vi "Begin.vi"(8 "error in":errorcluster) -> (0 "error out":errorcluster)   [LabVIEW 2017]
doc: "Called before other user functions, this VI is expected to open initial I/O refnums, load in file data, and do all program initialization. Notice that the <B>error out</B> terminal is simply used for data flow. Wiring it to other structures or subVIs ensures that this VI runs first."
uses:
  <vilib>/Rock Robotics/SystemInterfaces/DIO/FPGA_DIOPWMChannel.ctl
  <vilib>/Rock Robotics/WPI/SafetyOutput/WPI_SafetyOutputConfigMenu.ctl
  <vilib>/Rock Robotics/WPI/DriverStation/WPI_DriverStationRobotMode2.ctl
  <vilib>/Rock Robotics/WPI/Joystick/WPI_JoystickDeviceEnum.ctl
  <vilib>/Rock Robotics/SystemInterfaces/DIO/FPGA_DIOChannel.ctl
  <vilib>/Rock Robotics/SystemInterfaces/spilib/spi_bus.ctl
  <vilib>/Rock Robotics/WPI/RobotDrive/WPI_RobotDriveOpen2MotorWithVictorSP.vi
  Robot Global Data.vi
  <vilib>/Rock Robotics/Network Tables/NT Write String Array.vi
  <vilib>/Rock Robotics/WPI/Counter/WPI_CounterDigitalInputToDigitalSource.vi
  <vilib>/Rock Robotics/WPI/Gyro/WPI_GyroXRS450_SPI_Open.vi
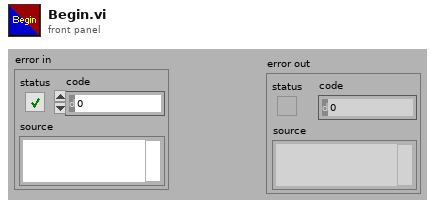
[diagram p1: front panel]
types:
  T1 = typedef "spi_bus.ctl" = enum16{"SPI On-Board, CS0", "SPI On-Board, CS1", "SPI On-Board, CS2", "SPI On-Board, CS3", "SPI MXP", "Invalid"}
  T2 = typedef "FPGA_DIOChannel.ctl" = enum8{"DIO 0", "DIO 1", "DIO 2", "DIO 3", "DIO 4", "DIO 5", "DIO 6", "DIO 7", "DIO 8", "DIO 9", "DIO MXP 0", "DIO MXP 1", "DIO MXP 2", "DIO MXP 3", "DIO MXP 4", "DIO MXP 5", "DIO MXP 6", "DIO MXP 7", "DIO MXP 8", "DIO MXP 9", "DIO MXP 10", "DIO MXP 11", "DIO MXP 12", "DIO MXP 13", "DIO MXP 14", "DIO MXP 15", "SPI Port CS1", "SPI Port CS2", "SPI Port CS3", "SPI Port MISO", "SPI Port MOSI", "Invalid"}
  T3 = typedef "WPI_JoystickDeviceEnum.ctl" = enum16{"USB 0", "USB 1", "USB 2", "USB 3", "USB 4", "USB 5"}
  T4 = typedef "WPI_DriverStationRobotMode2.ctl" = enum16{"Autonomous Disabled", "Autonomous Enabled", "Teleop Disabled", "Teleop Enabled", "Disconnected", "Finish", "Test Disabled", "Test Enabled", "Emergency Stopped"}
  T5 = typedef "WPI_SafetyOutputConfigMenu.ctl" = enum16{"Enable", "Disable"}
  T6 = typedef "FPGA_DIOPWMChannel.ctl" = enum8{"PWM 0", "PWM 1", "PWM 2", "PWM 3", "PWM 4", "PWM 5", "PWM 6", "PWM 7", "PWM 8", "PWM 9", "PWM MXP 0", "PWM MXP 1", "PWM MXP 2", "PWM MXP 3", "PWM MXP 4", "PWM MXP 5", "PWM MXP 6", "PWM MXP 7", "PWM MXP 8", "PWM MXP 9", "Invalid"}
  T7 = typedef "WPI_GyroDevRef.ctl" = cluster{"DevStatus":errorcluster, "Analog Channel":T8, "Gain (VoltsPerDegree/Second)":dbl, "Gyro Type":enum16{"Analog", "XRS450"}, "Handle":i32, "SPI Bus":T1, "Device Found":bool, "Sample Rate":dbl, "Calibrate On Open":bool, "Offset":dbl}
  T8 = typedef "FPGA_AIChannel.ctl" = enum8{"AI 0", "AI 1", "AI 2", "AI 3", "AI MXP 0", "AI MXP 1", "AI MXP 2", "AI MXP 3", "Invalid"}
  T9 = typedef "WPI_DigitalInputDevRef.ctl" = cluster{"DevStatus":errorcluster, "DIO Channel":T2}
  T10 = typedef "WPI_JoystickDevRef.ctl" = cluster{"Device":T3}
  T11 = typedef "WPI_RobotDriveDevRef.ctl" = cluster{"DevStatus":errorcluster, "Motors[]":T12[], "Square Inputs":bool, "Max Output":dbl}
  T12 = typedef "WPI_MotorControlDeviceRef.ctl" = cluster{"DeviceStatus":errorcluster, "Type":T13, "PWM":cluster{"PWM Channel":T6, "DeadBand":T14}, "CAN":cluster{"Device Number":u8, "SetOutput VI Ref":variant, "GetOutput VI Ref":variant, "Enable VI Ref":variant, "Disable VI Ref":variant, "Data":variant}, "Invert":bool, "DIO PWM":cluster{"PWM \"Enable\" Channel":T6, "DIOChannel":T2, "PWM Rate":dbl}}
  T13 = typedef "WPI_MotorControlType.ctl" = enum16{"PWM", "CAN", "DIO PWM"}
  T14 = typedef "WPI_PWMDeadband.ctl" = cluster{"Name":string, "maxPositivePwm":i32, "minPositivePwm":i32, "centerPwm":i32, "maxNegativePwm":i32, "minNegativePwm":i32, "angularRange":u16}
  T15 = typedef "FPGA_CounterEncoderSourceConvertionLVSourceType.ctl" = cluster{"DevStatus":errorcluster, "AnalogTriggerMode?":bool, "DigitalMode":cluster{"DIO Channel":T16}, "AnalogTriggerMode":cluster{"AnalogTriggerIndex":T17, "OutputType":T18}}
  T16 = typedef "FPGA_DIODigitalSourceChannel.ctl" = enum8{"DIO 0", "DIO 1", "DIO 2", "DIO 3", "DIO 4", "DIO 5", "DIO 6", "DIO 7", "DIO 8", "DIO 9", "DIO MXP 0", "DIO MXP 1", "DIO MXP 2", "DIO MXP 3", "DIO MXP 4", "DIO MXP 5", "DIO MXP 6", "DIO MXP 7", "DIO MXP 8", "DIO MXP 9", "DIO MXP 10", "DIO MXP 11", "DIO MXP 12", "DIO MXP 13", "DIO MXP 14", "DIO MXP 15", "Disabled"}
  T17 = typedef "FPGA_AnalogTriggerIndex.ctl" = enum8{"Trig 0", "Trig 1", "Trig 2", "Trig 3", "Trig 4", "Trig 5", "Trig 6", "Trig 7", "Invalid"}
  T18 = typedef "FPGA_AnalogTriggerOutType.ctl" = enum16{"InWindow", "TriggerState", "Rising", "Falling"}
  T19 = typedef "WPI_EncoderDevRef.ctl" = cluster{"DevStatus":errorcluster, "EncoderIndex":T20, "CounterIndex":T21, "DistancePerCount":dbl, "Decoding Type":T22}
  T20 = typedef "FPGA_EncoderIdx.ctl" = enum8{"Enc 0", "Enc 1", "Enc 2", "Enc 3", "Enc 4", "Enc 5", "Enc 6", "Enc 7", "Invalid"}
  T21 = typedef "FPGA_CounterCtrSystemIndex.ctl" = enum8{"Ctr 0", "Ctr 1", "Ctr 2", "Ctr 3", "Ctr 4", "Ctr 5", "Ctr 6", "Ctr 7", "Invalid"}
  T22 = typedef "WPI_EncoderType.ctl" = enum16{"1x", "2x", "4x"}
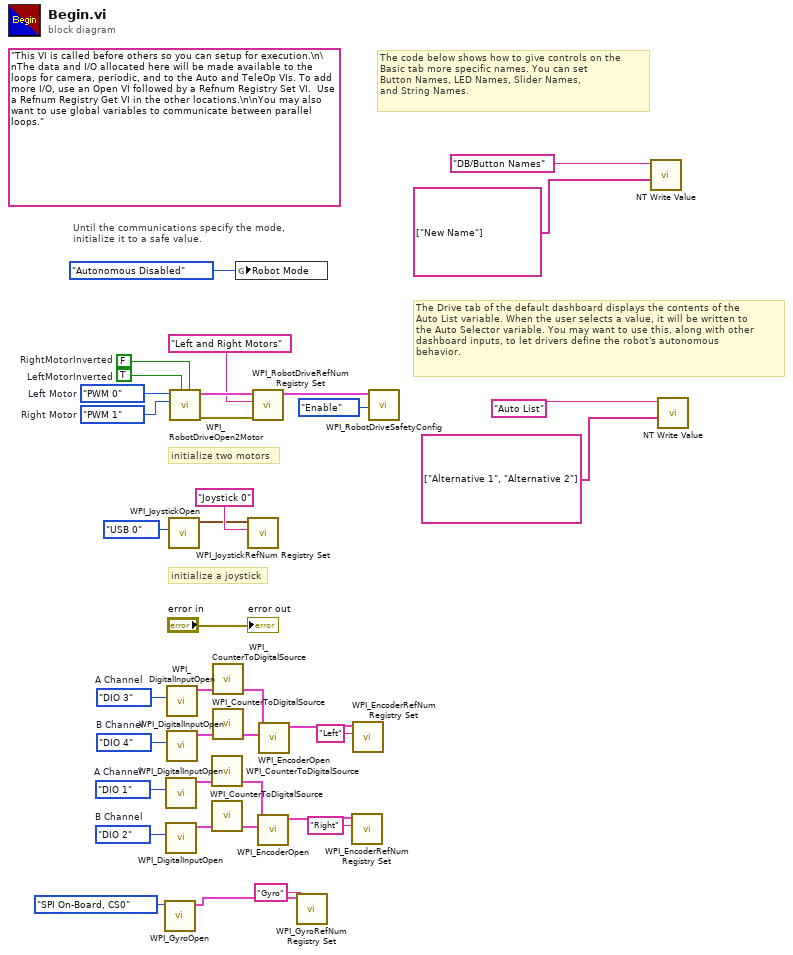
[diagram p0: block diagram]
diagram:
  w11 = FPGA_DIOChannel."DIO 2"  # B Channel
  w10 = FPGA_DIOChannel."DIO 1"  # A Channel
  w19 = FPGA_DIOChannel."DIO 4"  # B Channel
  w18 = FPGA_DIOChannel."DIO 3"  # A Channel
  (unwired) "This VI is called before others so you can setup for execution.\n\nThe data and I/O allocated here will be made available to the loops for camera, periodic, and to the Auto and TeleOp VIs. To add more I/O, use an Open VI followed by a Refnum Registry Set VI.  Use a Refnum Registry Get VI in the other locations.\n\nYou may also want to use global variables to communicate between parallel loops."
  w31 = FPGA_DIOPWMChannel."PWM 1"  # Right Motor
  w32 = FPGA_DIOPWMChannel."PWM 0"  # Left Motor
  w36 = TRUE  # LeftMotorInverted
  w37 = FALSE  # RightMotorInverted
  # "The Drive tab of the default dashboard displays the contents of the\nAuto List variable. When the user selects a value, it will be written to\nthe Auto Selector variable. You may want to use this, along with other\ndashboard inputs, to let drivers define the robot's autonomous\nbehavior."
  # "The code below shows how to give controls on the\nBasic tab more specific names. You can set\nButton Names, LED Names, Slider Names,\nand String Names."
  # "initialize a joystick"
  # "Until the communications specify the mode,\ninitialize it to a safe value."
  # "initialize two motors"
  n1 = call-poly <vilib>:"WPI_GyroOpen.vi"("SPI Bus"=spi_bus."SPI On-Board, CS0") -> ("GyroDevRef"=w2:T7)  [unwired: 8 in, 2 out]
  n2 = call <vilib>:"WPI_DigitalInputOpen.vi"("DIO Channel"=w10) -> ("DigitalInputDevRef"=w7:T9)  [unwired: 1 in, 9 out]
  n3 = call <vilib>:"WPI_DigitalInputOpen.vi"("DIO Channel"=w11) -> ("DigitalInputDevRef"=w8:T9)  [unwired: 1 in, 9 out]
  n4 = call <vilib>:"WPI_DigitalInputOpen.vi"("DIO Channel"=w18) -> ("DigitalInputDevRef"=w15:T9)  [unwired: 1 in, 9 out]
  n5 = call <vilib>:"WPI_DigitalInputOpen.vi"("DIO Channel"=w19) -> ("DigitalInputDevRef"=w16:T9)  [unwired: 1 in, 9 out]
  n6 = call <vilib>:"WPI_JoystickOpen.vi"("JoystickDevice"=WPI_JoystickDeviceEnum."USB 0") -> ("JoystickDevRef"=w26:T10)  [unwired: 10 in]
  n7 = call-poly <vilib>:"WPI_RobotDriveOpen2Motor.vi"("Right Motor Inverted"=w37, "Left Motor Inverted"=w36, "Right Motor"=w31, "Left Motor"=w32) -> ("error out"=w33:errorcluster, "RobotDriveDevRef"=w35:T11)  [unwired: 1 in, 5 out]
  n8 = call-poly <vilib>:"WPI_CounterToDigitalSource.vi"("DigitalInputDevRef"=w7) -> ("Digital Source"=w6:T15)  [unwired: 6 out]
  n9 = call-poly <vilib>:"WPI_CounterToDigitalSource.vi"("DigitalInputDevRef"=w8) -> ("Digital Source"=w9:T15)  [unwired: 6 out]
  n10 = call-poly <vilib>:"WPI_CounterToDigitalSource.vi"("DigitalInputDevRef"=w15) -> ("Digital Source"=w14:T15)  [unwired: 6 out]
  n11 = call-poly <vilib>:"WPI_CounterToDigitalSource.vi"("DigitalInputDevRef"=w16) -> ("Digital Source"=w17:T15)  [unwired: 6 out]
  n12 = global write "Robot Global Data.vi" "Robot Mode"(WPI_DriverStationRobotMode2."Autonomous Disabled" ("Robot Mode")) -> ()
  n13 = call <vilib>:"WPI_JoystickRefNum Registry Set.vi"("refnum name"="Joystick 0", "JoystickDevRef"=w26) -> ()  [unwired: 8 in, 2 out]
  n14 = call <vilib>:"WPI_RobotDriveRefNum Registry Set.vi"("error in (no error)"=w33, "refnum name"="Left and Right Motors", "RobotDriveDevRef"=w35) -> ("RobotDriveDevRef"=w30:T11)  [unwired: 1 in, 7 out]
  n15 = call <vilib>:"WPI_EncoderOpen.vi"("BSource"=w9, "ASource"=w6) -> ("EncoderDevRef"=w5:T19)  [unwired: 6 in, 3 out]
  n16 = call <vilib>:"WPI_EncoderOpen.vi"("BSource"=w17, "ASource"=w14) -> ("EncoderDevRef"=w13:T19)  [unwired: 6 in, 3 out]
  n17 = call <vilib>:"WPI_GyroRefNum Registry Set.vi"("refnum name"="Gyro", "GyroDevRef"=w2) -> ()  [unwired: 8 in, 2 out]
  n18 = call <vilib>:"WPI_EncoderRefNum Registry Set.vi"("refnum name"="Right", "EncoderDevRef"=w5) -> ()  [unwired: 8 in, 2 out]
  n19 = call <vilib>:"WPI_EncoderRefNum Registry Set.vi"("refnum name"="Left", "EncoderDevRef"=w13) -> ()  [unwired: 8 in, 2 out]
  n20 = call <vilib>:"WPI_RobotDriveSafetyConfig.vi"("mode"=WPI_SafetyOutputConfigMenu."Enable", "RobotDriveDevRef"=w30) -> ()  [unwired: 8 in, 2 out]
  n21 = call-poly <vilib>:"NT Write Value.vi"("String Array"=string[] ["New Name"], "Name"="DB/Button Names") -> ()  [unwired: 9 in, 1 out]
  n22 = call-poly <vilib>:"NT Write Value.vi"("String Array"=string[] ["Alternative 1", "Alternative 2"], "Name"="Auto List") -> ()  [unwired: 9 in, 1 out]
  "error out" <- "error in"
